vi "Stop Core.vi"(10 "final error code":i32, 11 "TopLevel in":refnum<class "TopLevel.lvclass">) -> (3 "TopLevel out":refnum<class "TopLevel.lvclass">)   [LabVIEW 2019, in "TopLevel.lvlib" / "TopLevel.lvclass"]
doc: "(<B>Filename</B>: Actor Framework.lvlib:Actor.lvclass:Stop Core.vi)\n\nDefines what the actor does before it stops. Use the <B>final error code</B> input to determine whether the actor shut down in response to an error.\n\nBy default, this method passes the Stop message along to all auto-stop nested actors. A descendant class may override this method to define additional behavior, such as shutting down any processes the actor initiated in its override of the Actor Core method."
uses:
  TopLevel.lvclass
  TopLevel.lvclass/TopLevel.ctl
  <vilib>/ActorFramework/Actor/Actor.lvclass
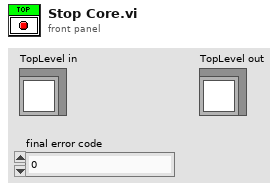
[diagram p1: front panel]
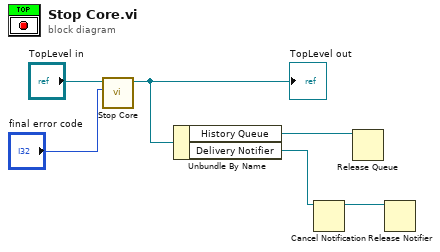
[diagram p0: block diagram]
diagram:
  n1 = call-parent "Stop Core.vi"("final error code"="final error code", "Actor in"="TopLevel in") -> ("Actor out"=w4:refnum<class "TopLevel.lvclass">)  [unwired: 9 in]
  "TopLevel out" <- w4
  n2 = Unbundle By Name(w4) -> ("History Queue"=w3:refnum<queue>, "Delivery Notifier"=w2:refnum<notifier>)
  n3 = Cancel Notification(0:w2) -> (8:w1:refnum<notifier>)  [unwired: 1 in, 2 out]
  n4 = Release Queue(queue=w3) -> ()  [unwired: 2 in, 3 out]
  n5 = Release Notifier(notifier=w1) -> ()  [unwired: 2 in, 3 out]
